vi "RGB to RGB565.vi"(8 "error in (no error)":errorcluster, 11 "Color in":refnum<class "Color.lvclass">) -> (0 "error out":errorcluster, 2 "Color":u16, 3 "Color out":refnum<class "Color.lvclass">)   [LabVIEW 2020, in "RPI.SenseHat.Display.lvlib" / "Color.lvclass"]
doc: "Converts the RGB888 to the RGB565 color."
uses:
  Color.lvclass
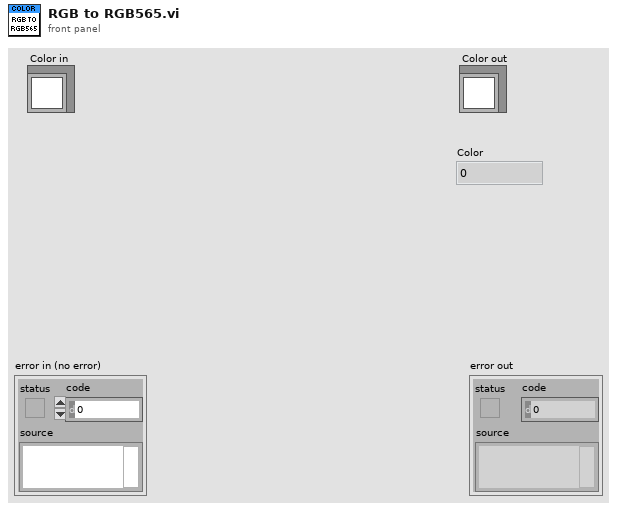
[diagram p1: front panel]
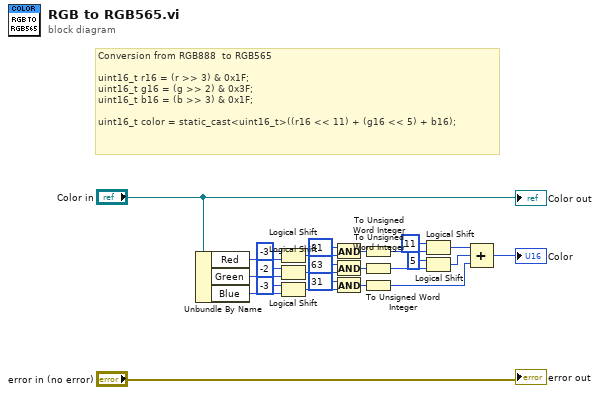
[diagram p0: block diagram]
diagram:
  # "Conversion from RGB888  to RGB565\n\nuint16_t r16 = (r >> 3) & 0x1F;\nuint16_t g16 = (g >> 2) & 0x3F;\nuint16_t b16 = (b >> 3) & 0x1F;\n\nuint16_t color = static_cast<uint16_t>((r16 << 11) + (g16 << 5) + b16);"
  n1 = Unbundle By Name("Color in") -> ("Red"=w4:u8, "Green"=w3:u8, "Blue"=w2:u8)
  n2 = Logical Shift(y=i16 -3, x=w4) -> (x << y=w8:u8)
  n3 = Logical Shift(y=i16 -2, x=w3) -> (x << y=w12:u8)
  n4 = Logical Shift(y=i16 -3, x=w2) -> (x << y=w13:u8)
  n5 = And(x=u8 31, y=w8) -> (x .and. y?=w15:u8)
  n6 = And(x=u8 63, y=w12) -> (x .and. y?=w17:u8)
  n7 = And(x=u8 31, y=w13) -> (x .and. y?=w20:u8)
  n8 = To Unsigned Word Integer(number=w15) -> (unsigned 16bit integer=w21:u16)
  n9 = To Unsigned Word Integer(number=w17) -> (unsigned 16bit integer=w22:u16)
  n10 = To Unsigned Word Integer(number=w20) -> (unsigned 16bit integer=w23:u16)
  n11 = Logical Shift(y=i16 11, x=w21) -> (x << y=w18:u16)
  n12 = Logical Shift(y=i16 5, x=w22) -> (x << y=w19:u16)
  n13 = Compound Arithmetic op=ADD(w18, w19, w23) -> (→"Color":u16)
  "error out" <- "error in (no error)"
  "Color out" <- "Color in"
